vi "construct.vi"(6 "cushion_model":T1 items=["Model 1", "Model 2"], 8 "error in (no error)":errorcluster, 9 "cost":dbl, 10 "id":u32) -> (0 "error out":errorcluster, 3 "Chair out":refnum<class "Chair.lvclass">)   [LabVIEW 2021, in "Chair.lvclass"]
uses:
  Chair.lvclass
  CushionModel.ctl
  Chair.lvclass/Chair.ctl
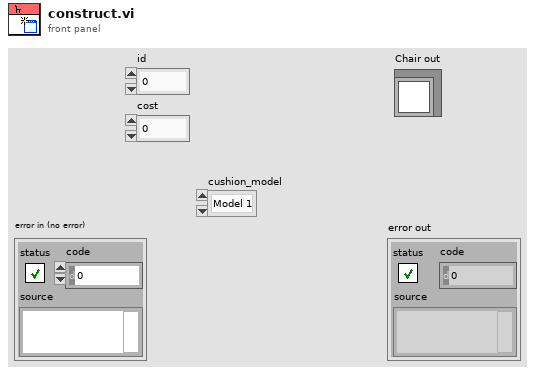
[diagram p1: front panel]
types:
  T1 = typedef "Chair.lvclass/CushionModel.ctl" = u16
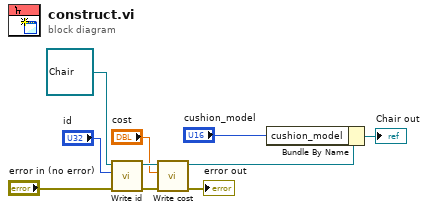
[diagram p0: block diagram]
diagram:
  n1 = call-dynamic "Write id.vi"("error in (no error)"="error in (no error)", "id"="id", "Furniture in"=refnum<class "Chair.lvclass"> refnum ("Chair.lvclass")) -> ("error out"=w6:errorcluster, "Furniture out"=w9:refnum<class "Chair.lvclass">)  [unwired: 7 in]
  n2 = call-dynamic "Write cost.vi"("error in (no error)"=w6, "price"="cost", "Furniture in"=w9) -> ("error out"=→"error out":errorcluster, "Furniture out"=w3:refnum<class "Chair.lvclass">)  [unwired: 7 in]
  n3 = Bundle By Name(cluster=w3, "cushion_model"="cushion_model") -> (→"Chair out":refnum<class "Chair.lvclass">)
